vi "DAQmx电压采集(单点).vi"(7 "被测通道":tag="PXI2Slot3/ai1", 8 "error in":errorcluster caption="错误输入", 11 "参考通道":tag="PXI2Slot3/ai0") -> (0 "error out":errorcluster caption="错误输出", 1 "被测幅值":dbl format="%.2p", 2 "参考幅值":dbl format="%.2p")   [LabVIEW 2015]
uses:
  <vilib>/Utility/error.llb/DialogType.ctl
  <vilib>/DAQmx/read.llb/DAQmx Read (Analog 1D Wfm NChan NSamp).vi
  <vilib>/DAQmx/create/channels.llb/DAQmx Create Channel (AI-Voltage-Basic).vi
  <vilib>/DAQmx/create/channels.llb/DAQmx Create Channel (AI-Acceleration-Accelerometer).vi
  <vilib>/DAQmx/configure/timing.llb/DAQmx Timing (Sample Clock).vi
  <vilib>/DAQmx/miscellaneous.llb/DAQmx Fill In Error Info.vi
  <vilib>/measure/matone.llb/Extract Single Tone Information N Chan.vi
  <resource>/objmgr/daqmx.rc
  <vilib>/measure/NI_MAPro.lvlib
panel:
  in  "停止":bool
  in  "IEPE":bool=TRUE
  in  "rate":dbl=1000.0 caption="速率" format="%0.2f"
  in  "samples per channel":i32=1000 caption="每通道采样"
  out "实际采样率":dbl=1000.0 format="%0.2f"
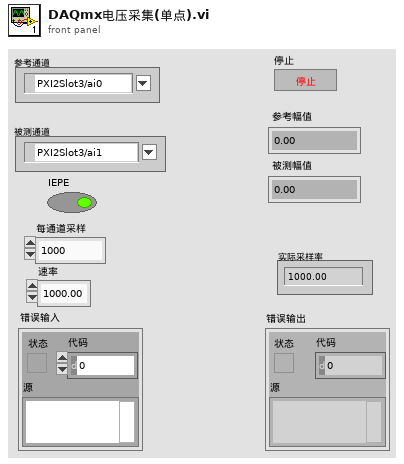
[diagram p1: front panel]
types:
  T1 = typedef "DialogType.ctl" = u16
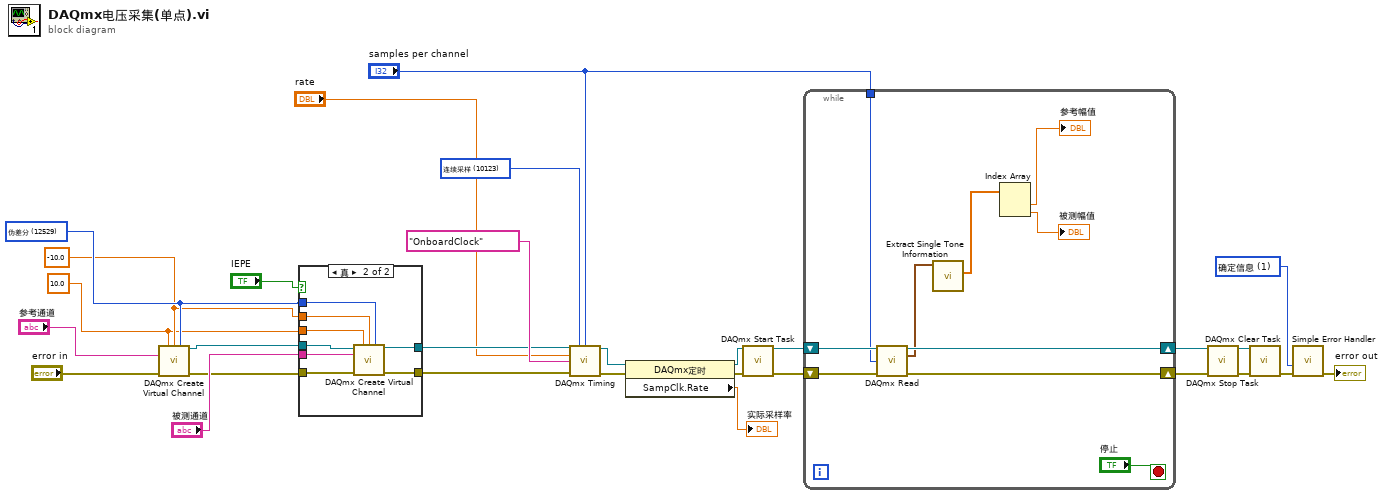
[diagram p0: block diagram]
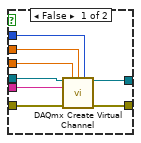
[diagram p2: hidden frame]
diagram:
  w18 = T1 1 items=["无对话框", "确定信息", "继续或停止信息", "确定信息＋警告", "继续/停止+警告"] ("type of dialog (OK msg:1)")
  w11 = 12529 items=["默认"=-1, "RSE"=10083, "NRSE"=10078, "差分"=10106, "伪差分"=12529] ("接线端配置")
  w9 = 10.0 ("最大电压")
  w10 = -10.0 ("最小电压")
  w29 = 10123 items=["有限采样"=10178, "连续采样"=10123, "硬件定时单点"=12522] ("sample mode")
  n1 = call-poly <vilib>:"DAQmx Create Virtual Channel.vi"("maximum value"=w9, "minimum value"=w10, "input terminal configuration"=w11, "physical channels"="参考通道", "error in"="error in") -> ("task out"=w5:refnum<k21>, "error out"=w7:errorcluster)  [unwired: 9 in]
  n2 = case shown="真" "IEPE" {
    tunnel: w11 -> [w37 w39]
    tunnel: w10 -> [w36 w40]
    tunnel: w9 -> [w35 w41]
    tunnel: w7 -> [w34 w44]
    tunnel: [w33 w42] -> w6
    tunnel: [w32 w43] -> w4
    tunnel: "被测通道" -> [w31 w45]
    tunnel: w5 -> [w30 w38]
    frame False {
      n3 = call-poly <vilib>:"DAQmx Create Virtual Channel.vi"("task in"=w30, "maximum value"=w35, "minimum value"=w36, "input terminal configuration"=w37, "physical channels"=w31, "error in"=w34) -> ("task out"=w32:refnum<k21>, "error out"=w33:errorcluster)  [unwired: 8 in]
    }
    frame True {
      n4 = call-poly <vilib>:"DAQmx Create Virtual Channel.vi"("task in"=w38, "maximum value"=w41, "minimum value"=w40, "input terminal configuration"=w39, "physical channels"=w45, "error in"=w44) -> ("task out"=w43:refnum<k21>, "error out"=w42:errorcluster)  [unwired: 8 in]
    }
  }
  n5 = call-poly <vilib>:"DAQmx Timing.vi"("task/channels in"=w4, "sample mode"=w29, "samples per channel"="samples per channel", "rate"="rate", "source"=tag "OnboardClock" ("采样时钟源"), "error in"=w6) -> ("task out"=w20:refnum<k21>, "error out"=w23:errorcluster)  [unwired: 8 in]
  n6 = property class="DAQmx定时"(reference=w20, error in=w23) -> (reference out=w24:refnum<k21>, error out=w22:errorcluster, "SampClk.Rate"=→"实际采样率":dbl)
  n7 = call <vilib>:"DAQmx Start Task.vi"("task/channels in"=w24, "error in"=w22) -> ("task out"=w12:refnum<k21>, "error out"=w13:errorcluster)  [unwired: 12 in]
  n8 = while {
    tunnel: "samples per channel" -> [w47]
    shift-right: [w54] -> w14
    shift-left: w13 -> [w53]
    shift-right: [w55] -> w17
    shift-left: w12 -> [w52]
    stop <- "停止" stop-if-true
    n9 = call-poly <vilib>:"DAQmx Read.vi"("task/channels in"=w52, "number of samples per channel"=w47, "error in"=w53) -> ("task out"=w55:refnum<k21>, "data"=w51:waveform(dbl)[], "error out"=w54:errorcluster)  [unwired: 10 in]
    n10 = call-poly <vilib>:"Extract Single Tone Information.vi"("time signals in"=w51) -> ("detected amplitudes"=w50:dbl[])  [unwired: 5 in, 5 out]
    n11 = Index Array(array=w50) -> (element #1=→"参考幅值":dbl, element #2=→"被测幅值":dbl)  [unwired: 2 in]
  }
  n12 = call <vilib>:"DAQmx Stop Task.vi"("task/channels in"=w17, "error in"=w14) -> ("task out"=w16:refnum<k21>, "error out"=w15:errorcluster)  [unwired: 12 in]
  n13 = call <vilib>:"DAQmx Clear Task.vi"("task in"=w16, "error in"=w15) -> ("error out"=w19:errorcluster)  [unwired: 13 in]
  n14 = call <vilib>:"Simple Error Handler.vi"("type of dialog (OK msg:1)"=w18, "error in (no error)"=w19) -> ("error out"=→"error out":errorcluster)  [unwired: 3 in, 4 out]
